vi "RSZVB Set Noise Figure Detector Measurement Time.vi"(8 "error in (no error)":errorcluster {"code" format="%.0x"}, 9 "Detector Time (0.01 s)":dbl=0.01 format="%^.3e", 10 "Channel (1)":i32=1, 11 "VISA session":refnum<visa-resource-name>) -> (0 "error out":errorcluster {"code" format="%.0x"}, 3 "dup VISA session":refnum<visa-resource-name>)   [LabVIEW 2011]
doc: "This VI sets the time that the analyzer uses to acquire data with each of the detector settings.\n\nNote(s):\n\n(1) This VI is available only with option R&S ZVAB-K30.\n\nRemote-control command(s):\n[SENSe<Ch>:]SWEep:DETector:TIME"
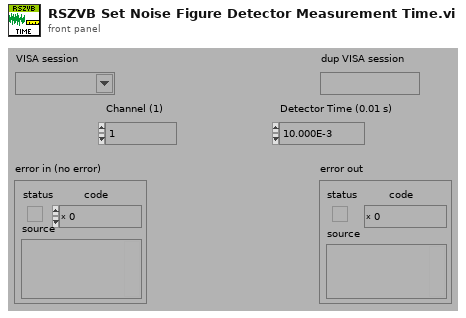
[diagram p1: front panel]
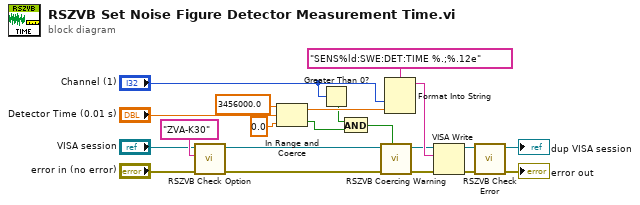
[diagram p0: block diagram]
diagram:
  n1 = call "RSZVB Check Option.vi"("error in (no error)"="error in (no error)", "Options"="ZVA-K30", "VISA session"="VISA session") -> ("error out"=w3:errorcluster, "dup VISA session"=w4:refnum<visa-resource-name>)  [unwired: 7 in]
  n2 = In Range and Coerce(upper limit=3456000.0, x="Detector Time (0.01 s)", lower limit=0.0) -> (coerced(x)=w12:dbl, In Range?=w8:bool)
  n3 = Greater Than 0?(x="Channel (1)") -> (x > 0?=w10:bool)
  n4 = And(x=w10, y=w8) -> (x .and. y?=w9:bool)
  n5 = call "RSZVB Coercing Warning.vi"("In Range?"=w9, "error in (no error)"=w3, "VISA session"=w4) -> ("error out"=w18:errorcluster, "dup VISA session"=w17:refnum<visa-resource-name>)  [unwired: 7 in]
  n6 = Format Into String(format string="SENS%ld:SWE:DET:TIME %.;%.12e", "Channel (1)", w12) -> (resulting string=w19:string)  [unwired: 2 in, 1 out]
  n7 = VISA Write(VISA resource name=w17, write buffer=w19, error in (no error)=w18) -> (VISA resource name out=w20:refnum<visa-resource-name>, error out=w21:errorcluster)  [unwired: 1 out]
  n8 = call "RSZVB Check Error.vi"("error in (no error)"=w21, "VISA session"=w20) -> ("error out"=→"error out":errorcluster, "dup VISA session"=→"dup VISA session":refnum<visa-resource-name>)  [unwired: 8 in]
